vi "Determine E-Series Membership.vi"(6 "Number of Bands":T3=4 min=3 max=6 step=1, 11 "E Serie":u16[](array[numeric])) -> (3 "In Serie?":bool)   [LabVIEW 2018]
doc: "Determines whether the resistance value obtained from the resistor digits belongs to the analyzed E-Series.\n\nThe VI receives the <b>E Series</b>, the <b>Resistance Digits</b>, and the <b>Number of Bands</b>. It uses <b>Build Resistor Cipher.vi</b> to build the corresponding cipher array and determines the resistance value represented by the resistor digits.\n\nThe resulting value is then searched in the values of the specified E-Series.\n\nThe VI returns <b>In Series?</b>, indicating whether the resistance value belongs to the analyzed E-Series."
uses:
  Number of Bands--number.ctl
  Resistance Digits--cluster.ctl
  Digit--enum.ctl
  Resistance Value/Resistance Value.lvlib
panel:
  in  "Resistance Digits":T1
  out "error out":errorcluster
  in  "error in (no error)":errorcluster
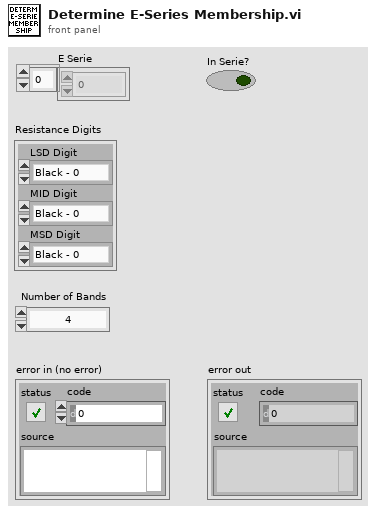
[diagram p1: front panel]
types:
  T1 = typedef "Resistance Digits--cluster.ctl" = cluster{"LSD Digit":T2, "MID Digit":T2, "MSD Digit":T2}
  T2 = typedef "digit--enum.ctl" = enum16{"Black - 0", "Brown - 1", "Red - 2", "Orange - 3", "Yellow - 4", "Green - 5", "Blue - 6", "Violet - 7", "Grey - 8", "White - 9"}
  T3 = typedef "Number of Bands--number.ctl" = u8
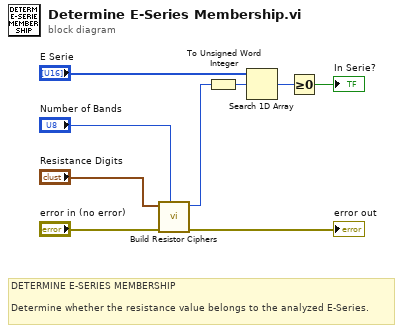
[diagram p0: block diagram]
diagram:
  # "DETERMINE E-SERIES MEMBERSHIP\n\nDetermine whether the resistance value belongs to the analyzed E-Series."
  n1 = call "Build Resistor Ciphers.vi"("Number of Bands"="Number of Bands", "error in (no error)"="error in (no error)", "Resistance Digits"="Resistance Digits") -> ("error out"=→"error out":errorcluster, "Nominal Value"=w6:i32)  [unwired: 6 in, 1 out]
  n2 = To Unsigned Word Integer(number=w6) -> (unsigned 16bit integer=w5:u16)
  n3 = Search 1D Array(1D array="E Serie", element=w5) -> (index of element=w8:i32)  [unwired: 1 in]
  n4 = Greater Or Equal To 0?(x=w8) -> (x >= 0?=→"In Serie?":bool)
